vi "Set View Status.vi"(8 "error in (no error)":errorcluster, 9 "View Status":T1, 10 "View":string, 11 "GUI Container in":refnum<class "GUI Container.lvclass">) -> (0 "error out":errorcluster, 2 "Status Added":bool, 3 "GUI Container out":refnum<class "GUI Container.lvclass">)   [LabVIEW 2023, in "GUI Views.lvlib" / "GUI Container.lvclass"]
uses:
  GUI Container.lvclass
  typedefs/View Status.ctl
  <vilib>/ActorFramework/Message Enqueuer/Message Enqueuer.lvclass
  typedefs/View Details.ctl
  typedefs/FP Status.ctl
  GUI Container.lvclass/GUI Container.ctl
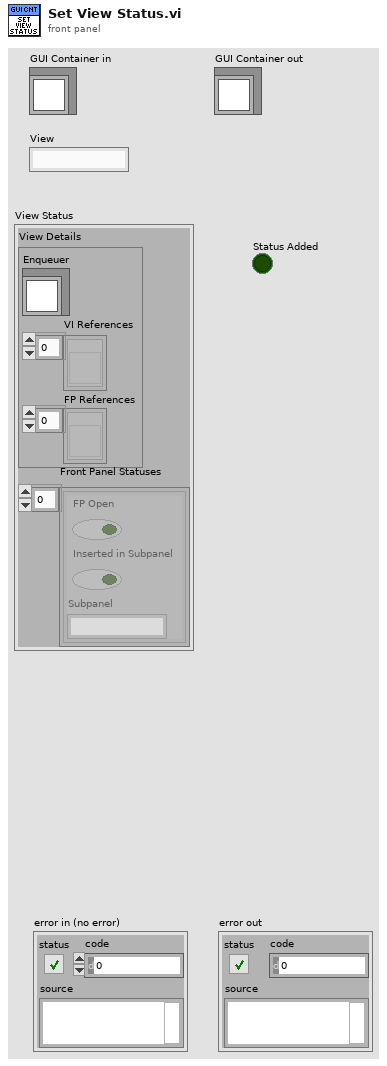
[diagram p1: front panel]
types:
  T1 = typedef "GUI Views.lvlib/GUI Container.lvclass/View Status.ctl" = cluster{"View Details":T2, "Front Panel Statuses":T3[]}
  T2 = typedef "GUI Views.lvlib/GUI Container.lvclass/View Details.ctl" = cluster{"Enqueuer":refnum<class "Message Enqueuer.lvclass">, "VI References":refnum<vi>[], "FP References":refnum<vi>[]}
  T3 = typedef "GUI Views.lvlib/GUI Container.lvclass/FP Status.ctl" = cluster{"FP Open":bool, "Inserted in Subpanel":bool, "Subpanel":string}
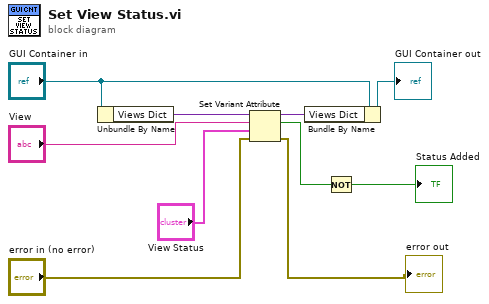
[diagram p0: block diagram]
diagram:
  n1 = Unbundle By Name("GUI Container in") -> ("Views Dict"=w4:variant)
  n2 = Set Variant Attribute(Variant=w4, name="View", value="View Status", error in="error in (no error)") -> (Variant out=w7:variant, replaced=w2:bool, error out=→"error out":errorcluster)
  n3 = Bundle By Name(cluster="GUI Container in", "Views Dict"=w7) -> (→"GUI Container out":refnum<class "GUI Container.lvclass">)
  n4 = Not(x=w2) -> (.not. x?=→"Status Added":bool)
